vi "Serial_Send.vi"(8 "error in":errorcluster, 9 "data":u8[](array[numeric]), 10 "messageID":u32) -> (0 "error out":errorcluster, 2 "sent data":u8[](array[numeric]))   [LabVIEW 2009, in "Serial.lvlib"]
doc: "Sends message to the serial port. To be used instead of sendMessage function from CAN Jaguar plug-in from FRC library."
uses:
  Serial.lvlib
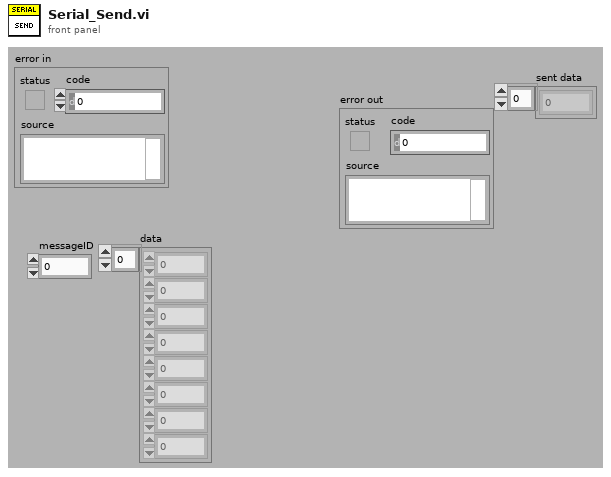
[diagram p1: front panel]
types:
  T1 = typedef "Semaphore RefNum" = refnum<k1>
  T2 = cluster{"VISA resource name":refnum<visa-resource-name>, "Semaphore":T1}
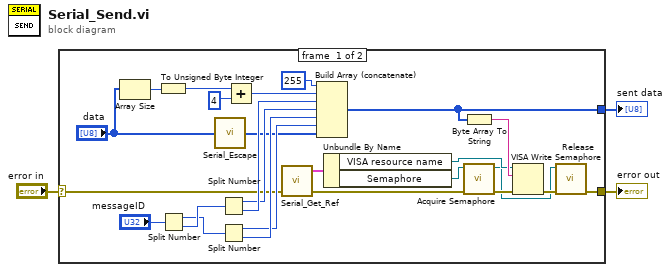
[diagram p0: block diagram]
diagram:
  n1 = case shown="No Error" "error in" {
    selector: "error in" -> [w15 w29]
    tunnel: [w9 w29] -> w3
    tunnel: [w16 _] -> w2
    frame #0 {
      n2 = Array Size(array="data") -> (size(s)=w6:i32)
      n3 = To Unsigned Byte Integer(number=w6) -> (unsigned 8bit integer=w28:u8)
      n4 = Split Number(x="messageID") -> (hi(x)=w23:u16, lo(x)=w24:u16)
      n5 = call "Serial_Escape.vi"("data"="data") -> ("data out"=w4:u8[])  [unwired: 4 in]
      n6 = Split Number(x=w24) -> (hi(x)=w19:u8, lo(x)=w20:u8)
      n7 = Split Number(x=w23) -> (hi(x)=w17:u8, lo(x)=w18:u8)
      n8 = Add(x=w28, y=u8 4) -> (x+y=w26:u8)
      n9 = call "Serial_Get_Ref.vi"("error in (no error)"=w15) -> ("error out"=w12:errorcluster, "Serial Ref"=w14:T2)  [unwired: 3 in]
      n10 = Build Array (concatenate)(u8 255 ("element"), w26, w20, w19, w18, w17, w4) -> (w16:u8[])
      n11 = Unbundle By Name(w14) -> ("VISA resource name"=w10:refnum<visa-resource-name>, "Semaphore"=w13:T1)
      n12 = Byte Array To String(unsigned byte array=w16) -> (string=w21:string)
      n13 = call <vilib>:"Acquire Semaphore.vi"("error in (no error)"=w12, "semaphore"=w13) -> ("error out"=w11:errorcluster, "semaphore out"=w7:T1)  [unwired: 3 in, 1 out]
      n14 = VISA Write(VISA resource name=w10, write buffer=w21, error in (no error)=w11) -> (error out=w8:errorcluster)  [unwired: 2 out]
      n15 = call <vilib>:"Release Semaphore.vi"("error in (no error)"=w8, "semaphore"=w7) -> ("error out"=w9:errorcluster)  [unwired: 4 in, 1 out]
    }
    frame #1 {
    }
  }
  "error out" <- w3
  "sent data" <- w2
